vi "Create Test Clusters.vi"(4 "error in":errorcluster) -> (0 "error out":errorcluster)   [LabVIEW 2025]
doc: "This VI creates all configured test Clusters for unit testing. The configuration file <i>Test Cluster Definition.xml</i> must lie in the same folder as this VI."
uses:
  Cluster Definition--cluster.ctl
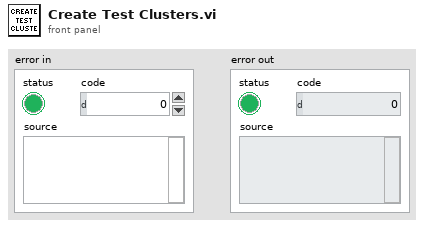
[diagram p1: front panel]
types:
  T1 = typedef "Cluster Definition--cluster.ctl" = cluster{"Name":string, "Description":string, "Numeric Indicators":cluster{"Labels":string[]}, "String Controls":cluster{"Labels":string[], "Default Values":string[]}, "Front Panel Labels":cluster{"Text":string[]}}
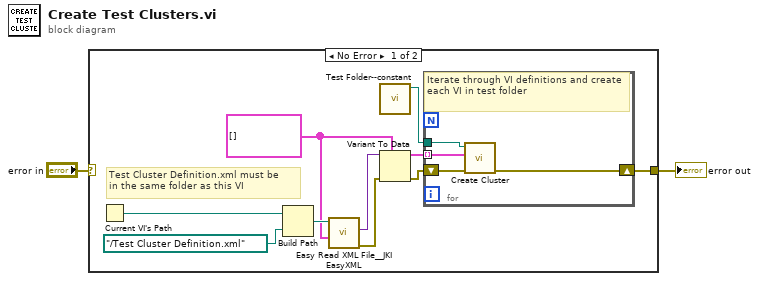
[diagram p0: block diagram]
diagram:
  n1 = case shown="No Error" "error in" {
    selector: "error in" -> [_ w17]
    tunnel: [w10 w17] -> w1
    frame No Error {
      w4 = T1[] [] ("Array")
      # "Test Cluster Definition.xml must be\nin the same folder as this VI"
      n2 = Current VI's Path() -> (path=w12:path)
      n3 = Build Path(base path=w12, name or relative path=path "../Test Cluster Definition.xml") -> (appended path=w7:path)
      n4 = call <vilib>:"Easy Read XML File__JKI EasyXML.vi"("LabVIEW Data (Type)"=w4, "XML File Path"=w7) -> ("error out"=w6:errorcluster, "LabVIEW Data"=w5:variant)  [unwired: 7 in, 1 out]
      n5 = call "Test Folder--constant.vi"() -> ("Test Folder"=w9:path)  [unwired: 7 in]
      n6 = Variant To Data(error in=w6, type=w4, Variant=w5) -> (data=w8:T1[], error out=w3:errorcluster)
      n7 = for {
        tunnel: w9 -> [w16]
        tunnel: w8 -> [w13] mode=indexing
        shift-right: [w14] -> w10
        shift-left: w3 -> [w15]
        # "Iterate through VI definitions and create each VI in test folder"
        n8 = call "Create Cluster.vi"("error in"=w15, "Cluster Definition"=w13, "Path"=w16) -> ("error out"=w14:errorcluster)  [unwired: 4 in]
      }
    }
    frame Error {
      # "Pass error without further action"
    }
  }
  "error out" <- w1
